vi "configureAcquisition_action.vi"(0 "HGF_ImaqDx":refnum<class "HGF_ImaqDx.lvclass">, 2 "Continuous?":enum16{"One-Shot", "Continuous"}(ring)=enum."Continuous", 3 "Number of buffers":u32, 5 "error in (no error)":errorcluster, 6 "Region of Interest":i32[](array[numeric]), 7 "Memory Location":enum16{"System", "Onboard"}(ring), 8 "Buffer Parameters":cluster{"Skip Count":u32, "Channel":i32}[](array[cluster]), 9 "Image Array":T1[](array[typedef])) -> (14 "dup HGF_ImaqDx":refnum<class "HGF_ImaqDx.lvclass">, 19 "error out":errorcluster)   [LabVIEW 2014, in "HGF_IMAQ.lvlib" / "HGF_ImaqDx.lvclass"]
doc: "Configures a low-level acquisition previously opened with IMAQdx Open Camera VI. Specify the acquisition type with the Continuous? and Number of Buffers parameters. \n\nSnap: Continuous = 0; Buffer Count = 1 \nSequence: Continuous = 0; Buffer Count > 1 \nGrab: Continuous = 1; Buffer Count > 1"
uses:
  HGF_ImaqDx.lvclass
  <vilib>/vision/driver/IMAQdx.llb/IMAQdx Acquisition Mode.ctl
  <vilib>/vision/Image Controls.llb/IMAQ Image.ctl
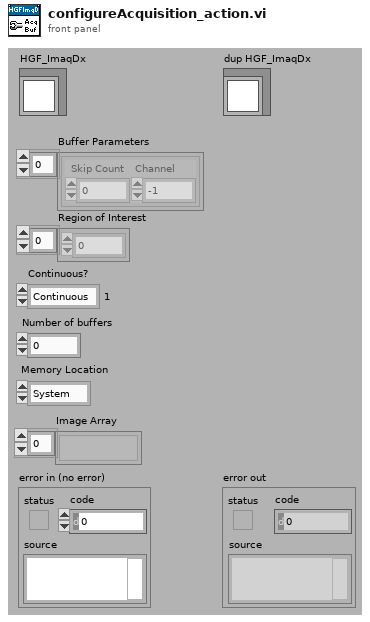
[diagram p1: front panel]
types:
  T1 = typedef "IMAQ Image.ctl" = refnum<image>
  T2 = typedef "NI_Vision_Acquisition_Software.lvlib/IMAQdx Acquisition Mode.ctl" = enum32{"One Shot", "Continuous"}
  T3 = typedef "IMAQdx.ctl" = refnum<k21>
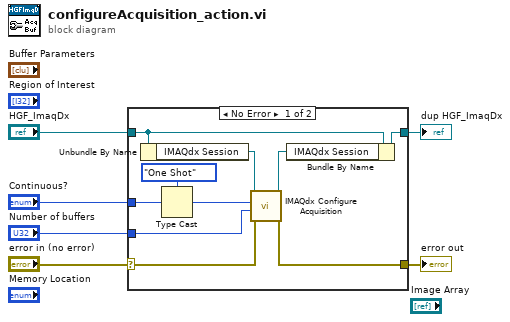
[diagram p0: block diagram]
diagram:
  n1 = case shown="No Error" "error in (no error)" {
    selector: "error in (no error)" -> [w7 w17]
    tunnel: "Continuous?" -> [w16 _]
    tunnel: "Number of buffers" -> [w13 _]
    tunnel: [w12 w17] -> w4
    tunnel: "HGF_ImaqDx" -> [w10 w18]
    tunnel: [w8 w18] -> w2
    frame No Error {
      n2 = Unbundle By Name(w10) -> ("IMAQdx Session"=w11:T3)
      n3 = Type Cast(type=IMAQdx_Acquisition_Mode."One Shot" ("Continuous?"), x=w16) -> (*(type *) &x=w14:T2)
      n4 = call <vilib>:"IMAQdx Configure Acquisition.vi"("error in"=w7, "Number of Buffers"=w13, "Continuous?"=w14, "Session In"=w11) -> ("error out"=w12:errorcluster, "Session Out"=w9:T3)  [unwired: 6 out]
      n5 = Bundle By Name(cluster=w10, "IMAQdx Session"=w9) -> (w8:refnum<class "HGF_ImaqDx.lvclass">)
    }
    frame Error {
    }
  }
  "error out" <- w4
  "dup HGF_ImaqDx" <- w2
